vi "Set UI VI Reference.vi"(8 "error in (no error)":errorcluster, 10 "UI VI Reference (caller)":refnum<vi>, 11 "Flex UI in":refnum<class "Flex UI.lvclass">) -> (0 "error out":errorcluster, 3 "Flex UI out":refnum<class "Flex UI.lvclass">)   [LabVIEW 2016, in "Flex UI.lvclass"]
doc: "Set the UI VI reference to the input VI reference if it is valid. If not use the calling VIs reference."
uses:
  Flex UI.lvclass
  Flex UI.lvclass/Flex UI.ctl
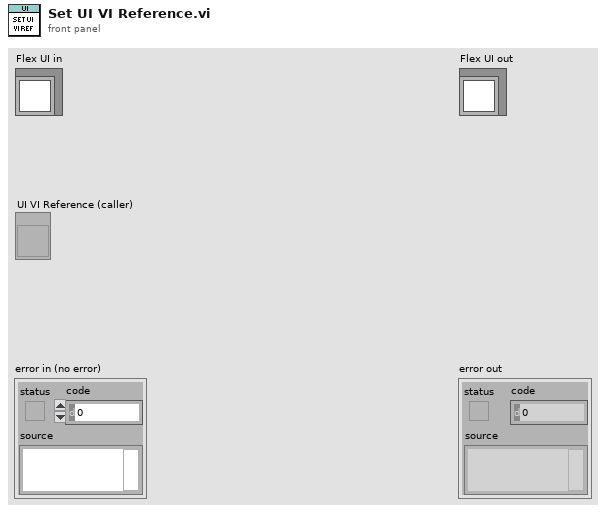
[diagram p1: front panel]
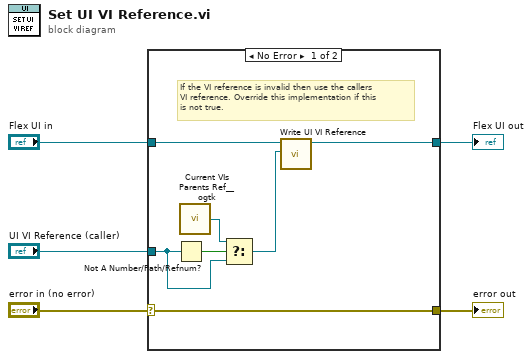
[diagram p0: block diagram]
diagram:
  n1 = case shown="No Error" "error in (no error)" {
    selector: "error in (no error)" -> [w11 w14]
    tunnel: [w11 w14] -> w4
    tunnel: [w10 w13] -> w2
    tunnel: "Flex UI in" -> [w12 w13]
    tunnel: "UI VI Reference (caller)" -> [w8 _]
    frame No Error {
      # "If the VI reference is invalid then use the callers\nVI reference. Override this implementation if this\nis not true."
      n2 = Not A Number/Path/Refnum?(number/path/refnum=w8) -> (NaN/Path/Refnum?=w9:bool)
      n3 = call <userlib>:"Current VIs Parents Ref__ogtk.vi"() -> ("Calling VI's Reference"=w7:refnum<vi>)  [unwired: 2 in]
      n4 = Select(t=w7, s=w9, f=w8) -> (s? t:f=w6:refnum<vi>)
      n5 = call "Write UI VI Reference.vi"("UI VI Reference"=w6, "Flex UI in"=w12) -> ("Flex UI out"=w10:refnum<class "Flex UI.lvclass">)  [unwired: 9 in]
    }
    frame Error {
    }
  }
  "error out" <- w4
  "Flex UI out" <- w2
